vi "ReadWriteLoopCase5.vi"() -> ()   [LabVIEW 2019]
uses:
  <vilib>/Platform/TimedLoop/XDataNode/timing_clust.ctl
  <vilib>/Platform/TimedLoop/XDataNode/nitl_modes.ctl
  <vilib>/Platform/TimedLoop/XDataNode/wakeup.ctl
  <vilib>/DAQmx/read.llb/DAQmx Read (Analog DBL 1Chan 1Samp).vi
  <vilib>/DAQmx/write.llb/DAQmx Write (Analog DBL 1Chan 1Samp).vi
  <vilib>/DAQmx/create/channels.llb/DAQmx Create Channel (AI-Voltage-Basic).vi
  <vilib>/DAQmx/create/channels.llb/DAQmx Create Channel (AO-Voltage-Basic).vi
  <vilib>/DAQmx/miscellaneous.llb/DAQmx Fill In Error Info.vi
  <vilib>/platform/TimedLoop/XDataNode/XDataNode.xnode
  <resource>/objmgr/daqmx.rc
  <vilib>/Platform/TimedLoop/XDataNode/XDNodeRunTimeDep.lvlib
panel:
  out "Finished Late? [i-1]":bool
  out "Actual End [i-1]":i64
  out "Expected End [i-1]":i64
  in  "stop":bool
  out "1/x":dbl
  out "Specified Write Rate":dbl
  out "Specified Sampling Rate":dbl
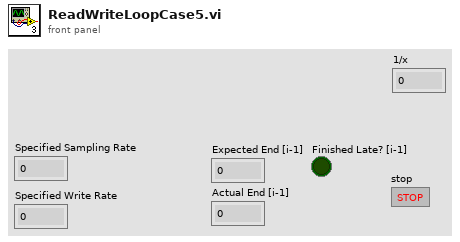
[diagram p1: front panel]
types:
  T1 = typedef "XDNodeRunTimeDep.lvlib/timing_clust.ctl" = cluster{"Expected End [f-1]":u64, "Actual End [f-1]":u64, "Finished Late? [f-1]":bool, "Expected End [i-1]":u64, "Actual End [i-1]":u64, "Finished Late? [i-1]":bool, "Expected Start [i]":u64, "Actual Start [i]":u64, "Expected Start [f]":u64, "Actual Start [f]":u64, "Source Name":string, "Structure Name":string, "Period":i64, "Deadline":i64, "Offset":i64, "Start":i64, "Priority":i32, "Timeout":i32, "Mode":T2, "Wakeup Reason":T3, "Error":errorcluster, "Source Type":string, "Secondary Source Type":string, "Global End Time":u64, "Global Start Time":u64, "Frame Duration":u64, "Iteration Duration":u64, "Assigned CPU":i32, "I/O Scan Engine Mode":u32}
  T2 = typedef "XDNodeRunTimeDep.lvlib/nitl_modes.ctl" = enum32{"No Change", "Process missed periods, maintain original phase", "Discard missed periods, maintain original phase", "Process missed periods, ignore original phase", "Discard missed periods, ignore original phase"}
  T3 = typedef "XDNodeRunTimeDep.lvlib/wakeup.ctl" = enum32{"Normal", "Aborted", "Asynchronous wakeup", "Timing source error", "Timed loop error", "Timeout"}
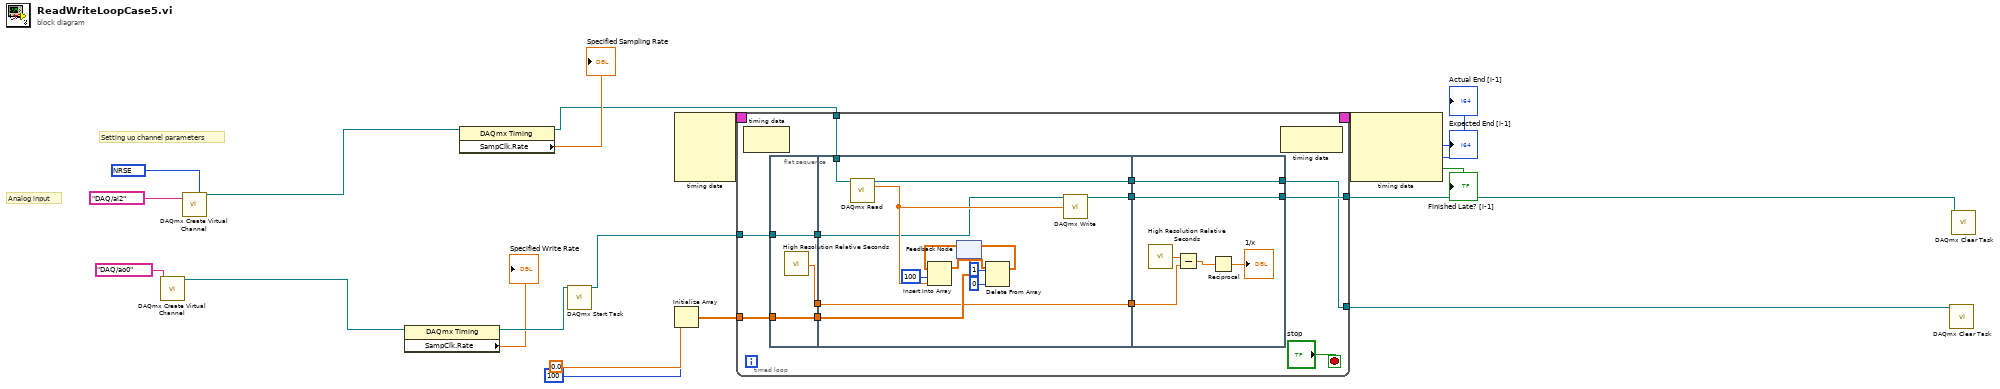
[diagram p0: block diagram]
diagram:
  w18 = 10078 items=["Default"=-1, "RSE"=10083, "NRSE"=10078, "Differential"=10106, "Pseudodifferential"=12529] ("input terminal configuration")
  # "Analog input"
  # "Setting up channel parameters"
  n1 = call-poly <vilib>:"DAQmx Create Virtual Channel.vi"("physical channels"=tag "DAQ/ao0") -> ("task out"=w1:refnum<k21>)  [unwired: 13 in, 1 out]
  n2 = call-poly <vilib>:"DAQmx Create Virtual Channel.vi"("input terminal configuration"=w18, "physical channels"=tag "DAQ/ai2") -> ("task out"=w3:refnum<k21>)  [unwired: 12 in, 1 out]
  n3 = property class="DAQmx Timing"(reference=w1) -> (reference out=w15:refnum<k21>, "SampClk.Rate"=→"Specified Write Rate":dbl)  [unwired: 1 in, 1 out]
  n4 = property class="DAQmx Timing"(reference=w3) -> (reference out=w2:refnum<k21>, "SampClk.Rate"=→"Specified Sampling Rate":dbl)  [unwired: 1 in, 1 out]
  n5 = call <vilib>:"DAQmx Start Task.vi"("task/channels in"=w15) -> ("task out"=w4:refnum<k21>)  [unwired: 13 in, 1 out]
  n6 = node-c288() -> (w20:T1)  [unwired: 4 in]
  n7 = Initialize Array(0.0 ("element"), 100 ("dimension size")) -> (w7:dbl[])
  n8 = timed-loop {
    timing: w20 -> [_]
    timing-out: [_] -> w19
    tunnel: w7 -> [w32]
    tunnel: [w30] -> w6
    tunnel: [w29] -> w5
    tunnel: w4 -> [w28]
    tunnel: w2 -> [w21]
    stop <- "stop" stop-if-true
    n9 = node-c288() -> ()  [unwired: 1 in, 1 out]
    n10 = flat-sequence {
      tunnel: w28 -> [w34]
      tunnel: w32 -> [w35]
      tunnel: [w35] -> w27
      tunnel: [w34] -> w26
      tunnel: [w33] -> w23
      tunnel: w27 -> [w41]
      tunnel: w26 -> [w38]
      tunnel: [w40] -> w25
      tunnel: [w39] -> w24
      tunnel: w23 -> [w37]
      tunnel: [w37] -> w22
      tunnel: w21 -> [w36]
      tunnel: [w53] -> w29
      tunnel: [w54] -> w30
      tunnel: w25 -> [w54]
      tunnel: w24 -> [w53]
      tunnel: w22 -> [w51]
      frame #0 {
        n11 = call <vilib>:"High Resolution Relative Seconds.vi"() -> ("relative seconds"=w33:dbl)
      }
      frame #1 {
        n12 = call-poly <vilib>:"DAQmx Read.vi"("task/channels in"=w36) -> ("task out"=w39:refnum<k21>, "data"=w48:dbl)  [unwired: 12 in, 1 out]
        n13 = feedback #1(w41) -> (w42:dbl[])
        n14 = Insert Into Array(array=w42, index=100, new element=w48) -> (w44:dbl[])
        n15 = Delete From Array(array=w44, length=1, index=0) -> (array with subset deleted=w43:dbl[])  [unwired: 1 out]
        n16 = feedback-in #1(w43) -> ()
        n17 = call-poly <vilib>:"DAQmx Write.vi"("task/channels in"=w38, "data"=w48) -> ("task out"=w40:refnum<k21>)  [unwired: 11 in, 2 out]
      }
      frame #2 {
        n18 = call <vilib>:"High Resolution Relative Seconds.vi"() -> ("relative seconds"=w52:dbl)
        n19 = Subtract(x=w52, y=w51) -> (x-y=w50:dbl)
        n20 = Reciprocal(x=w50) -> (1/x=→"1/x":dbl)
      }
    }
    n21 = node-c288() -> ()  [unwired: 1 in, 1 out]
  }
  n22 = node-c288(w19) -> (→"Expected End [i-1]":i64, →"Actual End [i-1]":i64, →"Finished Late? [i-1]":bool)  [unwired: 1 out]
  n23 = call <vilib>:"DAQmx Clear Task.vi"("task in"=w5) -> ()  [unwired: 14 in, 1 out]
  n24 = call <vilib>:"DAQmx Clear Task.vi"("task in"=w6) -> ()  [unwired: 14 in, 1 out]
